vi "File Status.vi"(6 "Data Path":path=path "C:/Data", 7 "ext":string=".bin", 8 "erriorIn":errorcluster, 9 "prefix":string, 10 "fSize":i64=50000000 caption="File Size (bytes)", 11 "fileRefIn":refnum<file>) -> (0 "error out":errorcluster, 3 "fileRefOut":refnum<file>)   [LabVIEW 2014, in "File Utilities.lvlib"]
uses:
  File Utilities.lvlib
panel:
  in  "nFile":bool
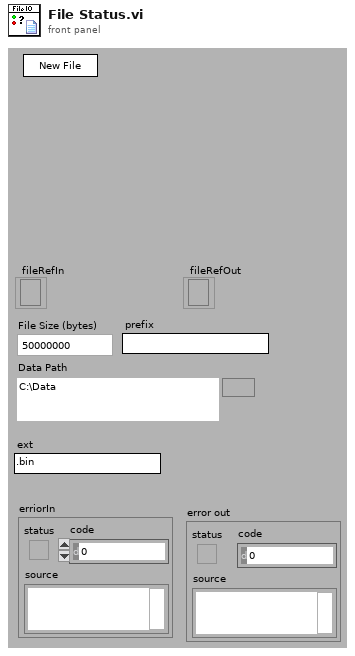
[diagram p1: front panel]
types:
  T1 = typedef "LVDateTimeRec.ctl" = cluster{"fractional second":dbl, "second":i32, "minute":i32, "hour":i32, "day of month":i32, "month":i32, "year":i32, "day of week":i32, "day of year":i32, "DST":i32}
  T2 = enum16{"open", "replace", "create", "open or create", "replace or create", "replace or create with confirmation"}
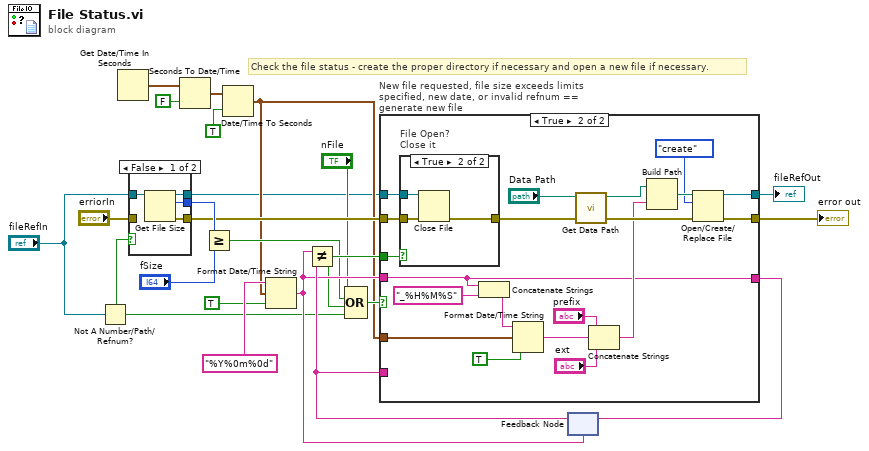
[diagram p0: block diagram]
diagram:
  # "Check the file status - create the proper directory if necessary and open a new file if necessary."
  n1 = Not A Number/Path/Refnum?(number/path/refnum="fileRefIn") -> (NaN/Path/Refnum?=w12:bool)
  n2 = Get Date/Time In Seconds() -> (seconds since 1Jan1904=w11:timestamp)
  n3 = case shown="False" w12 {
    tunnel: "fileRefIn" -> [w27 w29]
    tunnel: [w26 _] -> w17
    tunnel: [w25 w28] -> w15
    tunnel: [w24 w29] -> w3
    tunnel: "erriorIn" -> [_ w28]
    frame False {
      n4 = Get File Size(file=w27) -> (refnum out=w24:refnum<file>, size (in bytes)=w26:i64, 0:w25:errorcluster)  [unwired: 1 in]
    }
    frame True {
    }
  }
  n5 = Seconds To Date/Time(time stamp (now)=w11, to UTC (F)=FALSE) -> (date time rec=w8:T1)
  n6 = Greater Or Equal?(x=w17, y="fSize") -> (x >= y?=w14:bool)
  n7 = Date/Time To Seconds(1:TRUE ("is UTC (F)"), 2:w8) -> (0:w7:timestamp)
  n8 = Format Date/Time String(time format string (%c)="%Y%0m%0d", seconds (now)=w7, UTC format=TRUE) -> (date/time string=w20:string)
  n9 = feedback #1(w20) -> (w21:string)
  n10 = Not Equal?(x=w20, y=w21) -> (x != y?=w19:bool)
  n11 = Compound Arithmetic op=OR("nFile", w14, w19, w12) -> (w16:bool)
  n12 = case "New file requested, file size exceeds limits specified, new date, or invalid refnum == generate new file" shown="True" w16 {
    tunnel: [w32 w40] -> w23
    tunnel: w20 -> [_ w40]
    tunnel: w19 -> [_ w50]
    tunnel: [w31 w37] -> w1
    tunnel: w21 -> [w32 _]
    tunnel: w15 -> [w31 w48]
    tunnel: w7 -> [_ w42]
    tunnel: [w30 w38] -> w4
    tunnel: w3 -> [w30 w36]
    frame False {
    }
    frame True {
      n13 = case "File Open?\nClose it" shown="True" w50 {
        tunnel: [w53 w54] -> w34
        tunnel: w48 -> [w53 w56]
        tunnel: w36 -> [_ w55]
        frame False {
        }
        frame True {
          n14 = Close File(refnum=w55, error in=w56) -> (error out=w54:errorcluster)  [unwired: 1 out]
        }
      }
      n15 = Concatenate Strings(w40, "_%H%M%S" ("time format string (%c)")) -> (w44:string)
      n16 = Format Date/Time String(time format string (%c)=w44, seconds (now)=w42, UTC format=TRUE) -> (date/time string=w39:string)
      n17 = call "Get Data Path.vi"("error in"=w34, "Data Path In"="Data Path") -> ("error out"=w51:errorcluster, "Data Path Out"=w49:path)  [unwired: 8 in]
      n18 = Concatenate Strings("prefix", w39, "ext") -> (w46:string)
      n19 = Build Path(base path=w49, name or relative path=w46) -> (appended path=w52:path)
      n20 = Open/Create/Replace File(file path (use dialog)=w52, error in=w51, operation (0:open)=T2."create") -> (refnum out=w38:refnum<file>, error out=w37:errorcluster)  [unwired: 4 out]
    }
  }
  "fileRefOut" <- w4
  "error out" <- w1
  n21 = feedback-in #1(w23) -> ()
